vi "New Slider Position.vi"(8 "error in (no error)":errorcluster, 11 "Slider Ref Array":refnum<vi>[](array[refnum])) -> (0 "error out":errorcluster, 1 "Vertical Position Out":i32, 3 "Dup Slider Ref Array":refnum<vi>[](array[refnum]))   [LabVIEW 2020, in "3D Plot.lvclass"]
uses:
  3D Plot.lvclass
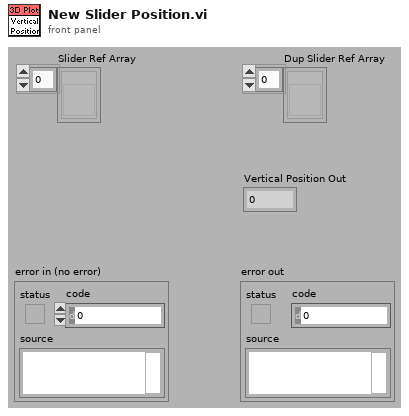
[diagram p1: front panel]
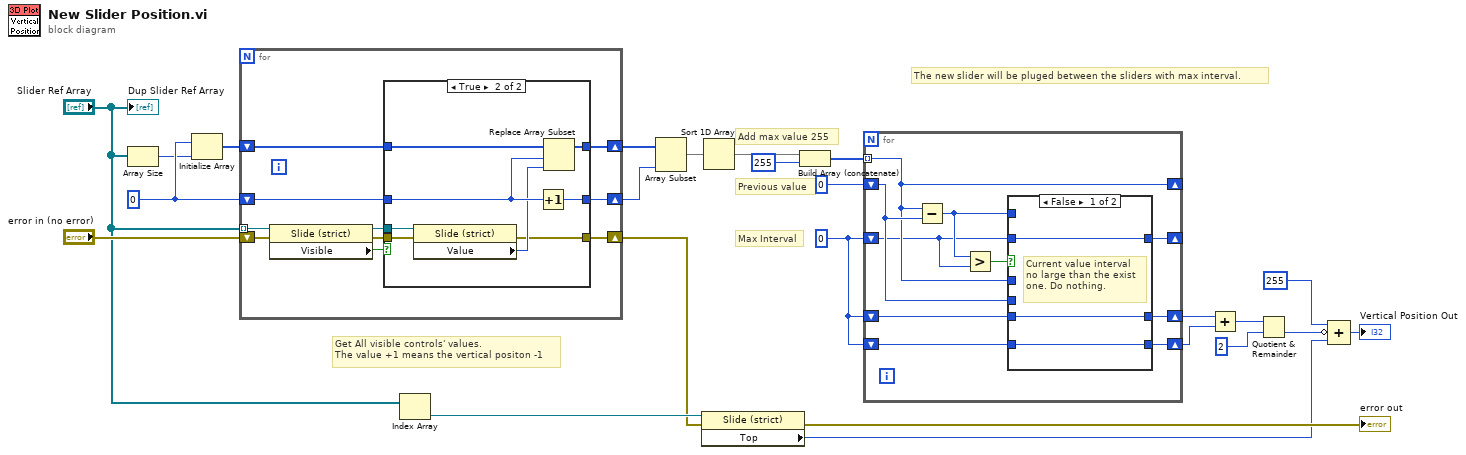
[diagram p0: block diagram]
diagram:
  w17 = 0
  w24 = 0
  # "The new slider will be pluged between the sliders with max interval."
  # "Add max value 255"
  # "Previous value"
  # "Max Interval"
  # "Get All visible controls' values. \nThe value +1 means the vertical positon -1"
  n1 = Array Size(array="Slider Ref Array") -> (size(s)=w22:i32)
  n2 = Initialize Array(w24, w22) -> (w23:i32[])
  n3 = for {
    tunnel: "Slider Ref Array" -> [w33] mode=indexing
    shift-right: [w32] -> w20
    shift-left: w24 -> [w31]
    shift-right: [w29] -> w21
    shift-left: w23 -> [w30]
    shift-right: [w25] -> w3
    shift-left: "error in (no error)" -> [w28]
    n4 = property class="Slide (strict)"(reference=w33, error in=w28) -> (reference out=w27:refnum<vi>, error out=w26:errorcluster, "Visible"=w34:bool)
    n5 = case shown="True" w34 {
      tunnel: [w36 w45] -> w32
      tunnel: w31 -> [w36 w42]
      tunnel: w30 -> [w37 w44]
      tunnel: [w37 w43] -> w29
      tunnel: w27 -> [_ w41]
      tunnel: w26 -> [w35 w39]
      tunnel: [w35 w38] -> w25
      frame False {
      }
      frame True {
        n6 = property class="Slide (strict)"(reference=w41, error in=w39) -> (error out=w38:errorcluster, "Value"=w40:i32)  [unwired: 1 out]
        n7 = Increment(x=w42) -> (x+1=w45:i32)
        n8 = Replace Array Subset(array=w44, new element=w40, index=w42) -> (w43:i32[])
      }
    }
  }
  n9 = Index Array(array="Slider Ref Array") -> (element=w7:refnum<vi>)  [unwired: 1 in]
  n10 = Array Subset(array=w21, length=w20) -> (w18:i32[])  [unwired: 1 in]
  n11 = property class="Slide (strict)"(reference=w7, error in=w3) -> (error out=→"error out":errorcluster, "Top"=w2:i32)  [unwired: 1 out]
  n12 = Sort 1D Array(array=w18) -> (sorted array=w11:i32[])
  n13 = Build Array (concatenate)(w11, 255 ("index")) -> (w9:i32[])
  n14 = for {
    tunnel: w9 -> [w49] mode=indexing
    shift-right: [w49] -> _
    shift-left: 0 ("index") -> [w50]
    shift-right: [w48] -> _
    shift-left: w17 -> [w46]
    shift-right: [w54] -> w16
    shift-left: w17 -> [w53]
    shift-right: [w52] -> w15
    shift-left: w17 -> [w51]
    n15 = Subtract(x=w49, y=w50) -> (x-y=w47:i32)
    n16 = Greater?(x=w47, y=w46) -> (0:w55:bool)
    n17 = case shown="False" w55 {
      tunnel: [w58 w61] -> w54
      tunnel: w53 -> [w58 _]
      tunnel: [w57 w60] -> w52
      tunnel: w51 -> [w57 _]
      tunnel: w49 -> [_ w61]
      tunnel: w50 -> [_ w60]
      tunnel: [w56 w59] -> w48
      tunnel: w47 -> [_ w59]
      tunnel: w46 -> [w56 _]
      frame False {
        # "Current value interval \nno large than the exist \none. Do nothing."
      }
      frame True {
        # "Save the largest \ninterval and its \ncorresponding\nvalues"
      }
    }
  }
  n18 = Add(x=w16, y=w15) -> (x+y=w14:i32)
  n19 = Quotient & Remainder(x=w14, y=2) -> (floor(x/y)=w5:i32)  [unwired: 1 out]
  n20 = Compound Arithmetic op=ADD(255 ("y"), invert w5, w2) -> (→"Vertical Position Out":i32)
  "Dup Slider Ref Array" <- "Slider Ref Array"
